vi "Initialize.vi"(8 "error in (no error)":errorcluster, 9 "Send \"Connect client\"":bool=TRUE, 10 "Reset":bool=TRUE, 11 "RP Instrument in":refnum<class "RP Instrument.lvclass">) -> (0 "error out":errorcluster, 3 "RP Instrument out":refnum<class "RP Instrument.lvclass">)   [LabVIEW 2018, in "RP Instrument.lvclass"]
uses:
  RP Instrument.lvclass
  RP Command.ctl
  RP Config Offsets.ctl
  RP Instrument.lvclass/RP Instrument.ctl
  RP Communicator/RP Communicator.lvclass
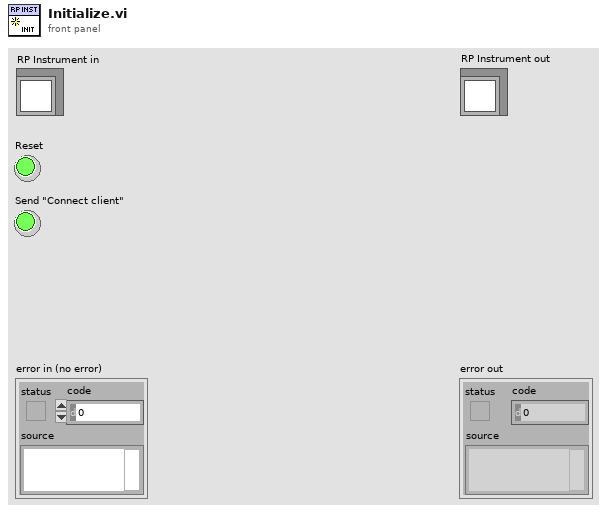
[diagram p1: front panel]
types:
  T1 = typedef "RP Config Offsets.ctl" = u16
  T2 = typedef "RP Command.ctl" = enum16{"Reset", "Read IDN", "Stop server", "Get status", "Get temperature", "Connect client", "Arm", "Software trigger", "Get whole buffer", "Get chunk", "System call", "Get config", "Set config", "Recieve data", "Recieve Calibartion", "Transmit data"}
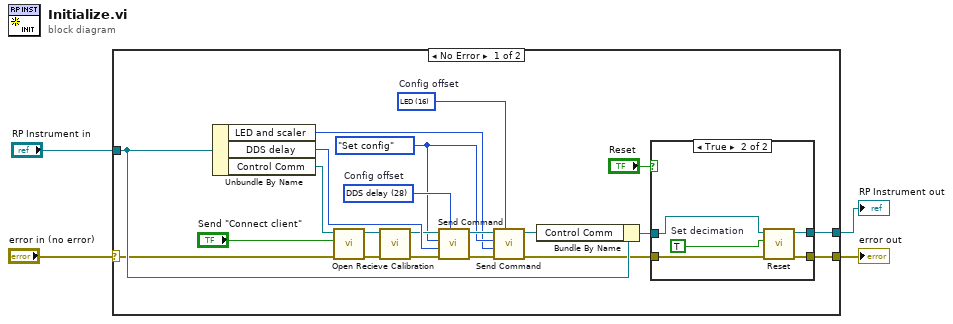
[diagram p0: block diagram]
diagram:
  n1 = case shown="No Error" "error in (no error)" {
    selector: "error in (no error)" -> [w23 w34]
    tunnel: [w6 w34] -> w3
    tunnel: [w7 w33] -> w1
    tunnel: "RP Instrument in" -> [w25 w33]
    frame No Error {
      w10 = T1 16 items=["Config flags"=0, "Record length"=4, "Frequency"=8, "Decimation"=12, "LED"=16, "DDS delay"=28]  # Config offset
      w20 = T1 28 items=["Config flags"=0, "Record length"=4, "Frequency"=8, "Decimation"=12, "LED"=16, "DDS delay"=28]  # Config offset
      w11 = RP_Command."Set config" ("Command number")
      n2 = Unbundle By Name(w25) -> ("LED and scaler"=w9:u32, "DDS delay"=w21:u32, "Control Comm"=w24:refnum<class "RP Communicator.lvclass">)
      n3 = call-dynamic "Open.vi"("error in (no error)"=w23, "Send \"Connect client\""="Send \"Connect client\"", "RP Communicator in"=w24) -> ("error out"=w16:errorcluster, "RP Communicator out"=w18:refnum<class "RP Communicator.lvclass">)  [unwired: 7 in]
      n4 = call-dynamic "Recieve Calibration.vi"("error in (no error)"=w16, "RP Communicator in"=w18) -> ("error out"=w15:errorcluster, "RP Communicator out"=w17:refnum<class "RP Communicator.lvclass">)  [unwired: 7 in, 1 out]
      n5 = call-dynamic "Send Command.vi"("Config offset"=w20, "error in (no error)"=w15, "Command payload"=w21, "Command number"=w11, "RP Communicator in"=w17) -> ("error out"=w12:errorcluster, "RP Communicator out"=w13:refnum<class "RP Communicator.lvclass">)  [unwired: 5 in]
      n6 = call-dynamic "Send Command.vi"("Config offset"=w10, "error in (no error)"=w12, "Command payload"=w9, "Command number"=w11, "RP Communicator in"=w13) -> ("error out"=w14:errorcluster, "RP Communicator out"=w5:refnum<class "RP Communicator.lvclass">)  [unwired: 5 in]
      n7 = Bundle By Name(cluster=w25, "Control Comm"=w5) -> (w8:refnum<class "RP Instrument.lvclass">)
      n8 = case shown="True" "Reset" {
        tunnel: [w26 w32] -> w6
        tunnel: w14 -> [w26 w29]
        tunnel: w8 -> [w27 w30]
        tunnel: [w27 w31] -> w7
        frame False {
        }
        frame True {
          w28 = TRUE  # Set decimation
          n9 = call-dynamic "Reset.vi"("error in (no error)"=w29, "Set decimation"=w28, "RP Instrument in"=w30) -> ("error out"=w32:errorcluster, "RP Instrument out"=w31:refnum<class "RP Instrument.lvclass">)  [unwired: 7 in]
        }
      }
    }
    frame Error {
    }
  }
  "error out" <- w3
  "RP Instrument out" <- w1
